vi "Get Listbox Row.vi"(8 "error in (no error)":errorcluster, 10 "Row":i32, 11 "MulticolumnListbox in":refnum<vi>) -> (0 "error out":errorcluster, 3 "Row Value":string[](array[string]))   [LabVIEW 2015, in "Diagnostics Addon System Explorer.lvlib"]
uses:
  Diagnostics Addon System Explorer.lvlib
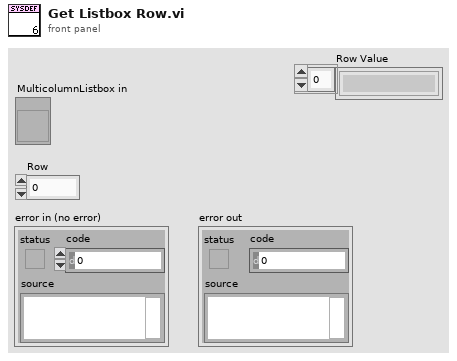
[diagram p1: front panel]
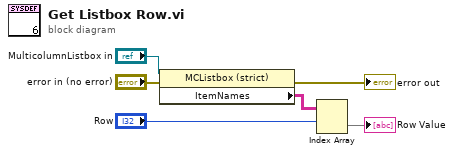
[diagram p0: block diagram]
diagram:
  n1 = property class="MCListbox (strict)"(reference="MulticolumnListbox in", error in="error in (no error)") -> (error out=→"error out":errorcluster, "ItemNames"=w4:string[][])  [unwired: 1 out]
  n2 = Index Array(array=w4, index (row)="Row") -> (element=→"Row Value":string[])  [unwired: 1 in]
